vi "Test Tokenizer Relative Single Command Formats.vi"(8 "error in (no error)":errorcluster) -> (0 "error out":errorcluster)   [LabVIEW 2019]
uses:
  PathTokenizer/PathTokenizer.lvclass
  PathTokenizer/PathTokenizer.lvclass/PathTokenizer.ctl
  <vilib>/addons/_JKI Toolkits/Caraya/classes/Assert/Assert Equal Value_Variant.vi
  <vilib>/addons/_JKI Toolkits/Caraya/classes/Assert/Assert.lvclass
  <vilib>/addons/_JKI Toolkits/Caraya/classes/Test/Test.lvclass
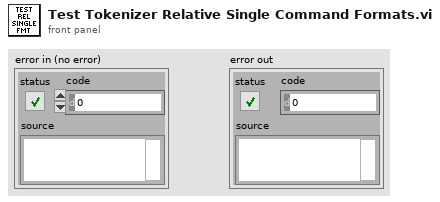
[diagram p1: front panel]
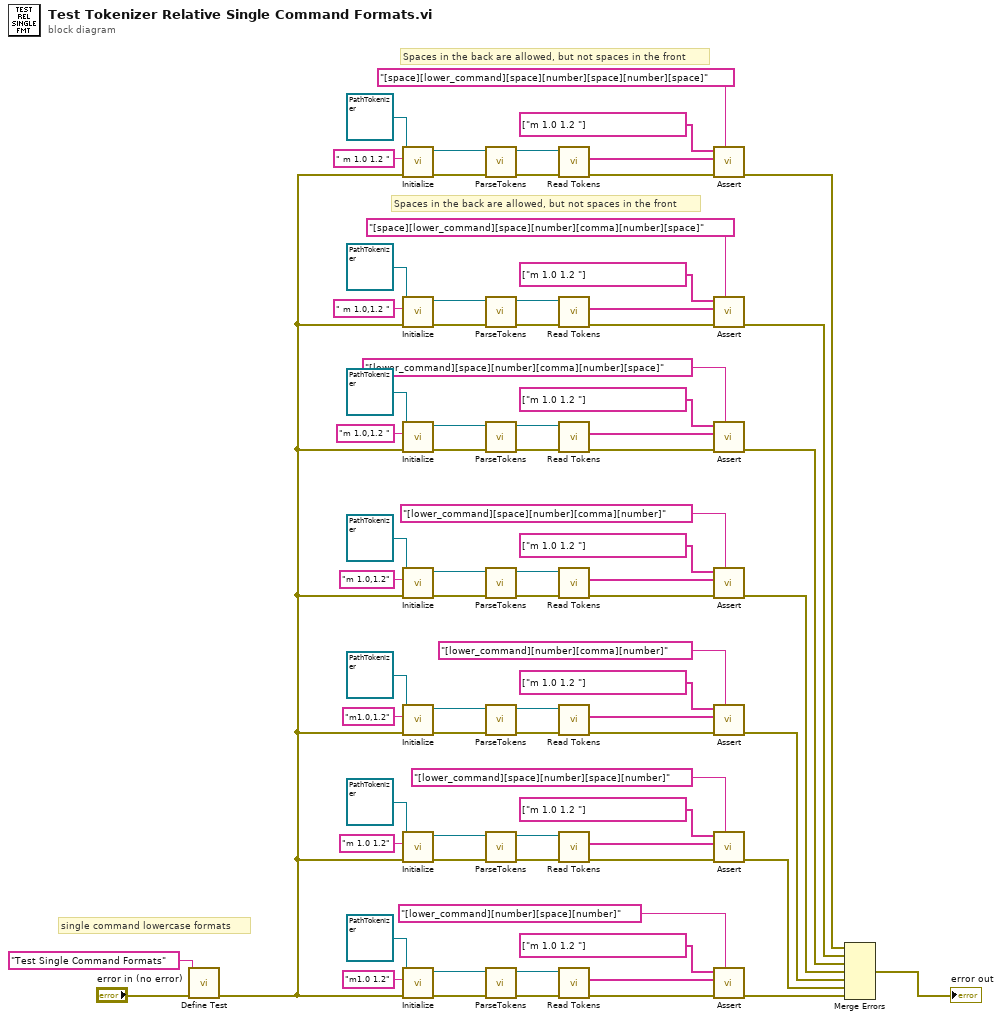
[diagram p0: block diagram]
diagram:
  # "Spaces in the back are allowed, but not spaces in the front"
  # "Spaces in the back are allowed, but not spaces in the front"
  # "single command lowercase formats"
  n1 = call <vilib>:"Define Test.vi"("error in (no error)"="error in (no error)", "Label (VI Title)"="Test Single Command Formats") -> ("error out"=w7:errorcluster)  [unwired: 8 in, 1 out]
  n2 = call "Initialize.vi"("error in (no error)"=w7, "Path Command Text"=" m 1.0 1.2 ", "PathTokenizer in"=refnum<class "PathTokenizer.lvclass"> refnum) -> ("error out"=w17:errorcluster, "PathTokenizer out"=w16:refnum<class "PathTokenizer.lvclass">)  [unwired: 7 in]
  n3 = call "Initialize.vi"("error in (no error)"=w7, "Path Command Text"=" m 1.0,1.2 ", "PathTokenizer in"=refnum<class "PathTokenizer.lvclass"> refnum) -> ("error out"=w18:errorcluster, "PathTokenizer out"=w19:refnum<class "PathTokenizer.lvclass">)  [unwired: 7 in]
  n4 = call "Initialize.vi"("error in (no error)"=w7, "Path Command Text"="m 1.0,1.2 ", "PathTokenizer in"=refnum<class "PathTokenizer.lvclass"> refnum) -> ("error out"=w37:errorcluster, "PathTokenizer out"=w36:refnum<class "PathTokenizer.lvclass">)  [unwired: 7 in]
  n5 = call "Initialize.vi"("error in (no error)"=w7, "Path Command Text"="m 1.0,1.2", "PathTokenizer in"=refnum<class "PathTokenizer.lvclass"> refnum) -> ("error out"=w39:errorcluster, "PathTokenizer out"=w40:refnum<class "PathTokenizer.lvclass">)  [unwired: 7 in]
  n6 = call "Initialize.vi"("error in (no error)"=w7, "Path Command Text"="m1.0,1.2", "PathTokenizer in"=refnum<class "PathTokenizer.lvclass"> refnum) -> ("error out"=w58:errorcluster, "PathTokenizer out"=w57:refnum<class "PathTokenizer.lvclass">)  [unwired: 7 in]
  n7 = call "Initialize.vi"("error in (no error)"=w7, "Path Command Text"="m 1.0 1.2", "PathTokenizer in"=refnum<class "PathTokenizer.lvclass"> refnum) -> ("error out"=w59:errorcluster, "PathTokenizer out"=w60:refnum<class "PathTokenizer.lvclass">)  [unwired: 7 in]
  n8 = call "Initialize.vi"("error in (no error)"=w7, "Path Command Text"="m1.0 1.2", "PathTokenizer in"=refnum<class "PathTokenizer.lvclass"> refnum) -> ("error out"=w79:errorcluster, "PathTokenizer out"=w78:refnum<class "PathTokenizer.lvclass">)  [unwired: 7 in]
  n9 = call "ParseTokens.vi"("error in (no error)"=w17, "PathTokenizer in"=w16) -> ("error out"=w12:errorcluster, "PathTokenizer out"=w13:refnum<class "PathTokenizer.lvclass">)  [unwired: 8 in]
  n10 = call "ParseTokens.vi"("error in (no error)"=w18, "PathTokenizer in"=w19) -> ("error out"=w23:errorcluster, "PathTokenizer out"=w22:refnum<class "PathTokenizer.lvclass">)  [unwired: 8 in]
  n11 = call "ParseTokens.vi"("error in (no error)"=w37, "PathTokenizer in"=w36) -> ("error out"=w32:errorcluster, "PathTokenizer out"=w33:refnum<class "PathTokenizer.lvclass">)  [unwired: 8 in]
  n12 = call "ParseTokens.vi"("error in (no error)"=w39, "PathTokenizer in"=w40) -> ("error out"=w44:errorcluster, "PathTokenizer out"=w43:refnum<class "PathTokenizer.lvclass">)  [unwired: 8 in]
  n13 = call "ParseTokens.vi"("error in (no error)"=w58, "PathTokenizer in"=w57) -> ("error out"=w53:errorcluster, "PathTokenizer out"=w54:refnum<class "PathTokenizer.lvclass">)  [unwired: 8 in]
  n14 = call "ParseTokens.vi"("error in (no error)"=w59, "PathTokenizer in"=w60) -> ("error out"=w64:errorcluster, "PathTokenizer out"=w63:refnum<class "PathTokenizer.lvclass">)  [unwired: 8 in]
  n15 = call "ParseTokens.vi"("error in (no error)"=w79, "PathTokenizer in"=w78) -> ("error out"=w74:errorcluster, "PathTokenizer out"=w75:refnum<class "PathTokenizer.lvclass">)  [unwired: 8 in]
  n16 = call "Read Tokens.vi"("error in (no error)"=w12, "PathTokenizer in"=w13) -> ("error out"=w9:errorcluster, "Tokens"=w11:string[])  [unwired: 7 in, 1 out]
  n17 = call "Read Tokens.vi"("error in (no error)"=w23, "PathTokenizer in"=w22) -> ("error out"=w26:errorcluster, "Tokens"=w24:string[])  [unwired: 7 in, 1 out]
  n18 = call "Read Tokens.vi"("error in (no error)"=w32, "PathTokenizer in"=w33) -> ("error out"=w29:errorcluster, "Tokens"=w31:string[])  [unwired: 7 in, 1 out]
  n19 = call "Read Tokens.vi"("error in (no error)"=w44, "PathTokenizer in"=w43) -> ("error out"=w47:errorcluster, "Tokens"=w45:string[])  [unwired: 7 in, 1 out]
  n20 = call "Read Tokens.vi"("error in (no error)"=w53, "PathTokenizer in"=w54) -> ("error out"=w50:errorcluster, "Tokens"=w52:string[])  [unwired: 7 in, 1 out]
  n21 = call "Read Tokens.vi"("error in (no error)"=w64, "PathTokenizer in"=w63) -> ("error out"=w67:errorcluster, "Tokens"=w65:string[])  [unwired: 7 in, 1 out]
  n22 = call "Read Tokens.vi"("error in (no error)"=w74, "PathTokenizer in"=w75) -> ("error out"=w71:errorcluster, "Tokens"=w73:string[])  [unwired: 7 in, 1 out]
  n23 = call-poly <vilib>:"Assert.vi"("Label"="[space][lower_command][space][number][space][number][space]", "error in (no error)"=w9, "Y"=w11, "X"=string[] ["m 1.0 1.2 "] ("Tokens")) -> ("error out"=w1:errorcluster)  [unwired: 6 in, 1 out]
  n24 = call-poly <vilib>:"Assert.vi"("Label"="[space][lower_command][space][number][comma][number][space]", "error in (no error)"=w26, "Y"=w24, "X"=string[] ["m 1.0 1.2 "] ("Tokens")) -> ("error out"=w2:errorcluster)  [unwired: 6 in, 1 out]
  n25 = call-poly <vilib>:"Assert.vi"("Label"="[lower_command][space][number][comma][number][space]", "error in (no error)"=w29, "Y"=w31, "X"=string[] ["m 1.0 1.2 "] ("Tokens")) -> ("error out"=w3:errorcluster)  [unwired: 6 in, 1 out]
  n26 = call-poly <vilib>:"Assert.vi"("Label"="[lower_command][space][number][comma][number]", "error in (no error)"=w47, "Y"=w45, "X"=string[] ["m 1.0 1.2 "] ("Tokens")) -> ("error out"=w4:errorcluster)  [unwired: 6 in, 1 out]
  n27 = call-poly <vilib>:"Assert.vi"("Label"="[lower_command][number][comma][number]", "error in (no error)"=w50, "Y"=w52, "X"=string[] ["m 1.0 1.2 "] ("Tokens")) -> ("error out"=w5:errorcluster)  [unwired: 6 in, 1 out]
  n28 = call-poly <vilib>:"Assert.vi"("Label"="[lower_command][space][number][space][number]", "error in (no error)"=w67, "Y"=w65, "X"=string[] ["m 1.0 1.2 "] ("Tokens")) -> ("error out"=w6:errorcluster)  [unwired: 6 in, 1 out]
  n29 = call-poly <vilib>:"Assert.vi"("Label"="[lower_command][number][space][number]", "error in (no error)"=w71, "Y"=w73, "X"=string[] ["m 1.0 1.2 "] ("Tokens")) -> ("error out"=w69:errorcluster)  [unwired: 6 in, 1 out]
  n30 = Merge Errors(w1, w2, w3, w4, w5, w6, w69) -> (→"error out":errorcluster)
